vi "dfd_LatticeAllpass_Basic_IIR_C.vi"() -> ()   [LabVIEW 2017, in "NI_DigFilterTemp.lvlib"]
uses:
  <vilib>/addons/Digital Filter Design/NI_DigFilterTemp.lvlib
panel:
  in  "String":string="\n\n/* ---- Constants ----*/\n#define %CapName%_N_STATES %kIIRStatesAmt%\n#define %CapName%_N_COEFK %CapName%_N_STATES\n\n/* ---- Global Variables Declaration ----*/\nstatic %CoefAType% %FilterBlkName%_CoefK[%CapName%_N_COEFK];\n%InternalFunctionsDeclaration%\n\n%ShiftDefine%\n\n%AssistantFunctions%\n\n/* ---- Implement the Fixed-Point Filter ---- */ \n%OutType% %FilterBlkName%_Filtering (%InType% sampleIn, %FilterBlkName%_State state)\n{\n\tI32 accA, accB;\n\t%MultType% mult;\n\tint i;\n\t\n\taccB = (%I32TypeCast%sampleIn << IN2SUM);\n\n\t/* Filtering */\n\tfor (i=0; i < %CapName%_N_STATES; i++)\n\t{\n\t\tmult = %PreMultCast%(state[i] << DELAY2MULT);\n\t\taccB -= (%FilterBlkName%_%MultA%(mult, %FilterBlkName%_CoefK[i]) << PROD2SUM);\n\t\tmult = %PreMultCast%(accB << SUM2MULT);\n\t\taccA = (%FilterBlkName%_%MultA%(mult, %FilterBlkName%_CoefK[i]) << PROD2SUM);\n\t\taccA += (state[i] << DELAY2SUM);\n\t\tstate[i] = accA;\n\t}\n\taccA = state[0];\n\n\t/* Update the internal states */\n\tfor (i=0; i < %CapName%_N_STATES-1; i++)\n\t\tstate[i] = (state[i+1] << SUM2DELAY);\n\tstate[i] = (accB << SUM2DELAY);\n\t\n\t%ApplyGainAccA%\n\n\treturn (%OutType%)accA;\n}\n\n/* ---- Internal Functions ---- */\n%InternalFunctions%\n\n/* ---- Filter Coefficients ---- */\nstatic %CoefAType% %FilterBlkName%_CoefK [] = {\n%CoefficientsK%\n};\n"
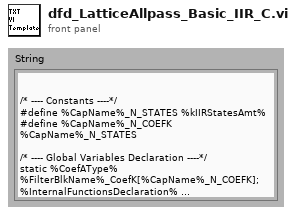
[diagram p1: front panel]
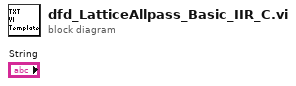
[diagram p0: block diagram]
diagram:
